vi "test_csm_helper2.vi"() -> ()   [LabVIEW 2020]
uses:
  <vilib>/Utility/traverseref.llb/TRef TravTarget.ctl
  <userlib>/_NEVSTOP/Communicable State Machine(CSM)/_Support/Priority Queue/Priority Queue.lvclass/Priority Queue.ctl
  Properties/Read VI Ref.vi
  <userlib>/_NEVSTOP/Communicable State Machine(CSM)/Utility/Build Error Cluster.vi
  <userlib>/_NEVSTOP/Communicable State Machine(CSM)/_Support/Process/CSMP-Sync Call.vi
  <userlib>/_NEVSTOP/Communicable State Machine(CSM)/Utility/uuid.vi
  <userlib>/_NEVSTOP/Communicable State Machine(CSM)/Utility/Trim Both Whitespace.vi
  <userlib>/_NEVSTOP/Communicable State Machine(CSM)/_Support/Process/CSMP-Async Call.vi
  <userlib>/_NEVSTOP/Communicable State Machine(CSM)/_Support/GlobalEvent/GEvt-Generate Status Log.vi
  <userlib>/_NEVSTOP/Communicable State Machine(CSM)/_Support/Process/CSMP-Broadcast.vi
  <userlib>/_NEVSTOP/Communicable State Machine(CSM)/_Support/GlobalEvent/GEvt-Generate Interrupt Log.vi
  <userlib>/_NEVSTOP/Communicable State Machine(CSM)/_Support/GlobalEvent/GEvt-Generate Register Log.vi
  <userlib>/_NEVSTOP/Communicable State Machine(CSM)/_Support/Process/CSMP-Register Status.vi
  <userlib>/_NEVSTOP/Communicable State Machine(CSM)/_Support/GlobalEvent/GEvt-Generate Unregister Log.vi
  <userlib>/_NEVSTOP/Communicable State Machine(CSM)/_Support/Process/CSMP-Unregister Status.vi
  <userlib>/_NEVSTOP/Communicable State Machine(CSM)/_Support/CSMQ/_CSMObj-Unlock.vi
  <userlib>/_NEVSTOP/Communicable State Machine(CSM)/_Support/Process/CSMP-PostPostMsg.vi
  <userlib>/_NEVSTOP/Communicable State Machine(CSM)/_Support/Process/CSMP-PostSendMsg.vi
  <userlib>/_NEVSTOP/Communicable State Machine(CSM)/_Support/CSMQ/_CSMObj-Lock State.vi
  <userlib>/_NEVSTOP/Communicable State Machine(CSM)/_Support/Common/Splite Reason String Part.vi
  <userlib>/_NEVSTOP/Communicable State Machine(CSM)/_Support/Common/Trim Single line Text.vi
  <userlib>/_NEVSTOP/Communicable State Machine(CSM)/_Support/CSMQ/_CSMOFGV Release.vi
  <userlib>/_NEVSTOP/Communicable State Machine(CSM)/_Support/Common/Remove Comments from Line.vi
  <userlib>/_NEVSTOP/Communicable State Machine(CSM)/_Support/Common/Splite Single-line Message.vi
  <userlib>/_NEVSTOP/Communicable State Machine(CSM)/_Support/Common/Parse Next Single-line State.vi
  <userlib>/_NEVSTOP/Communicable State Machine(CSM)/_Support/CSMQ/_CSMOFGV Dequeue.vi
  <userlib>/_NEVSTOP/Communicable State Machine(CSM)/_Support/CSMQ/_CSMObj-Log Error if in a Remote Session.vi
  <userlib>/_NEVSTOP/Communicable State Machine(CSM)/_Support/GlobalEvent/GEvt-Generate State Change Log.vi
  <userlib>/_NEVSTOP/Communicable State Machine(CSM)/_Support/GlobalEvent/GEvt-Generate Remaining States Log.vi
  <userlib>/_NEVSTOP/Communicable State Machine(CSM)/_Support/GlobalEvent/GEvt-Generate Module Destroyed Log.vi
  <userlib>/_NEVSTOP/Communicable State Machine(CSM)/_Support/GlobalEvent/GEvt-Generate Complete Log.vi
  <userlib>/_NEVSTOP/Communicable State Machine(CSM)/_Support/GlobalEvent/GEvt-Generate Module Created Log.vi
  <userlib>/_NEVSTOP/Communicable State Machine(CSM)/AdvanceAPI/CSM - Revert Arguments-Safe String.vi
  <userlib>/_NEVSTOP/Communicable State Machine(CSM)/AdvanceAPI/CSM - Make String Arguments Safe.vi
  <userlib>/_NEVSTOP/Communicable State Machine(CSM)/_Support/CSMQ/_CSMObj-Message Check.vi
  <userlib>/_NEVSTOP/Communicable State Machine(CSM)/_Support/CSMQ/_CSMObj-Enqueue Cross-Module Message.vi
  <userlib>/_NEVSTOP/Communicable State Machine(CSM)/_Support/CSMQ/_CSMOFGV Get.vi
  <userlib>/_NEVSTOP/Communicable State Machine(CSM)/_Support/FGV-BroadcastRegistry/Cache-Broadcast Registry Search Result.vi
  <userlib>/_NEVSTOP/Communicable State Machine(CSM)/AdvanceAPI/CSM - Register Status Change.vi
  <userlib>/_NEVSTOP/Communicable State Machine(CSM)/AdvanceAPI/CSM - Unregister Status Change.vi
  <userlib>/_NEVSTOP/Communicable State Machine(CSM)/_Support/Common/Hex Str to U8 Data.vi
  <userlib>/_NEVSTOP/Communicable State Machine(CSM)/_Support/Common/Concatenate State with Arguments.vi
  <userlib>/_NEVSTOP/Communicable State Machine(CSM)/_Support/Common/U8 Data to Hex Str.vi
  <userlib>/_NEVSTOP/Communicable State Machine(CSM)/_Support/Priority Queue/Dequeue Element.vi
  <userlib>/_NEVSTOP/Communicable State Machine(CSM)/AdvanceAPI/CSM - Keywords.vi
  <userlib>/_NEVSTOP/Communicable State Machine(CSM)/_Support/Priority Queue/Enqueue Element.vi
  <userlib>/_NEVSTOP/Communicable State Machine(CSM)/_Support/GlobalEvent/FGV-GlobalEventRef.vi
  <userlib>/_NEVSTOP/Communicable State Machine(CSM)/_Support/CSMQ/_CSMOFGV Obtain.vi
  <userlib>/_NEVSTOP/Communicable State Machine(CSM)/_Support/CSMQ/_CSMOFGV.vi
  <userlib>/_NEVSTOP/Communicable State Machine(CSM)/_Support/GlobalEvent/FGV-StatusChangeEventRef.vi
  <userlib>/_NEVSTOP/Communicable State Machine(CSM)/_Support/FGV-BroadcastRegistry/global-CSMQ FGV Change Flag.vi
  <userlib>/_NEVSTOP/Communicable State Machine(CSM)/_Support/FGV-BroadcastRegistry/global-Broadcast Cache Change Flag.vi
  <userlib>/_NEVSTOP/Communicable State Machine(CSM)/_Support/BroadcastRegistry/HelperVI/Broadcast Item Key.vi
  <userlib>/_NEVSTOP/Communicable State Machine(CSM)/_Support/FGV-BroadcastRegistry/FGV-BroadcastRegistry.vi
  <userlib>/_NEVSTOP/Communicable State Machine(CSM)/_Support/Message/Parse Register Message.vi
  <userlib>/_NEVSTOP/Communicable State Machine(CSM)/_Support/Message/Parse Unregister Message.vi
  API/Create From VI Reference.vi
  API/Destroy.vi
  <userlib>/_NEVSTOP/Communicable State Machine(CSM)/Communicable State Machine.lvlib
  CSM-Helper.lvclass
  <vilib>/Utility/traverseref.llb/VI Scripting - Traverse.lvlib
  34952832-c283-4153-b183-f70f505a0969.vi
panel:
  out "Array":path[](array[path])
  out "State History":string
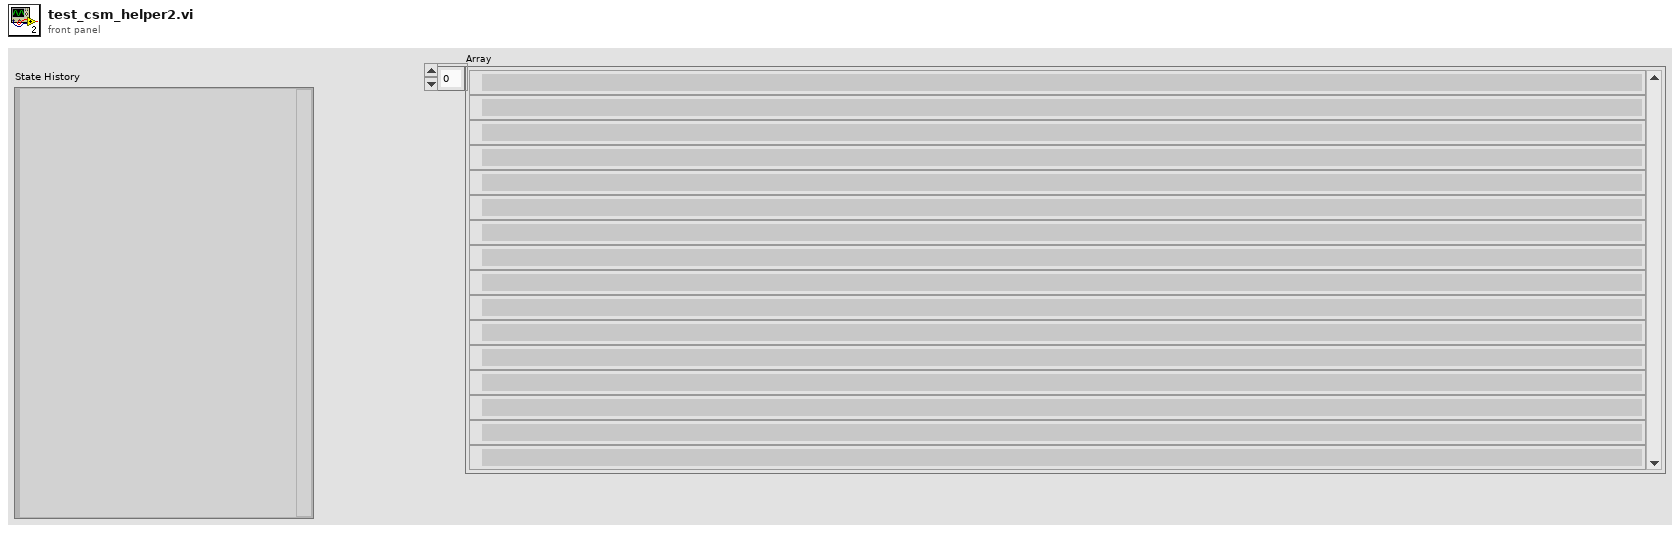
[diagram p1: front panel]
types:
  T1 = typedef "TRef TravTarget.ctl" = enum16{"FP", "BD", "Other"}
  T2 = enum32{"Invalid", "Standard", "Closed", "Hidden", "Minimized", "Maximized"}
  T3 = enum32{"invalid app kind", "Development System", "Run Time System", "Student Edition", "Embedded LabVIEW", "Evaluation", "Custom"}
  T4 = typedef "Communicable State Machine.lvlib/_CSM_Response Source Message.ctl" = cluster{"‘State":string, "’Arguments":string, "’Error":errorcluster}
  T5 = cluster{"Core":cluster{"Current VI Reference":refnum<vi>, "Close Panel on Exit?":bool}, "Your Boolean data":bool, "Your string data":string}
  T6 = cluster{"Current VI Reference":refnum<vi>, "Close Panel on Exit?":bool}
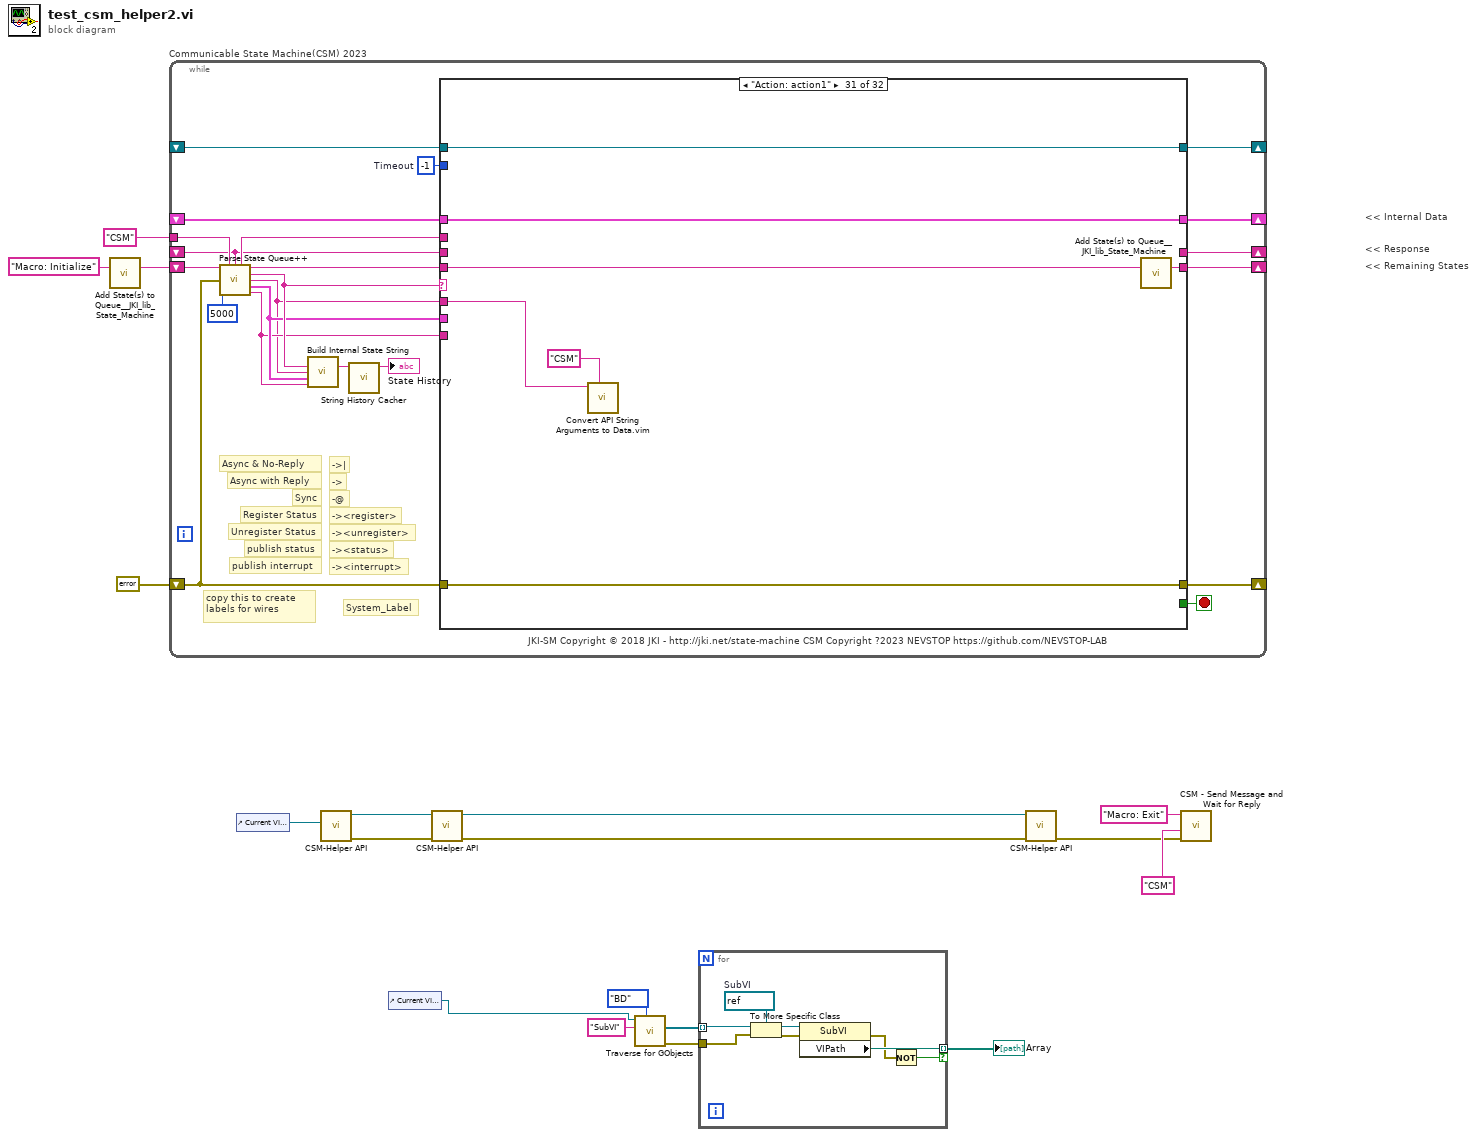
[diagram p0: block diagram]
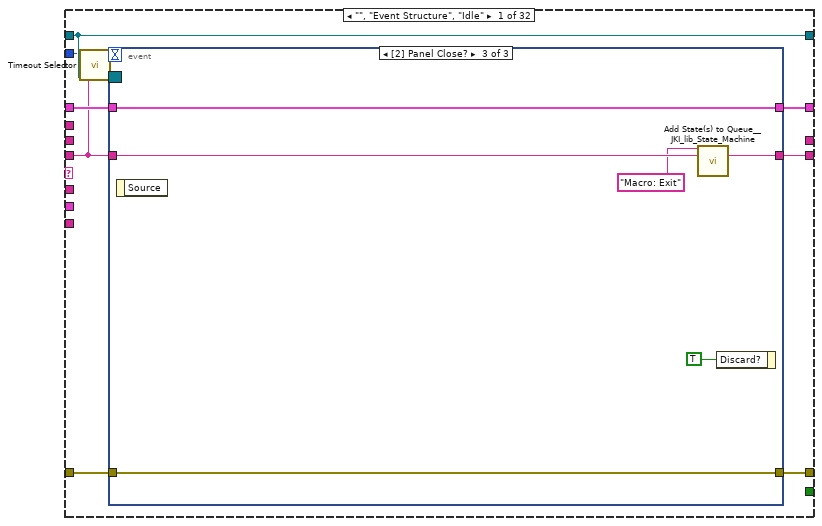
[diagram p2: hidden frame]
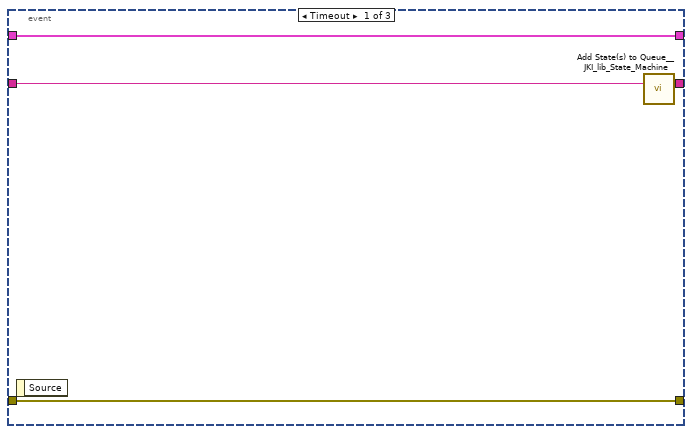
[diagram p3: hidden frame]
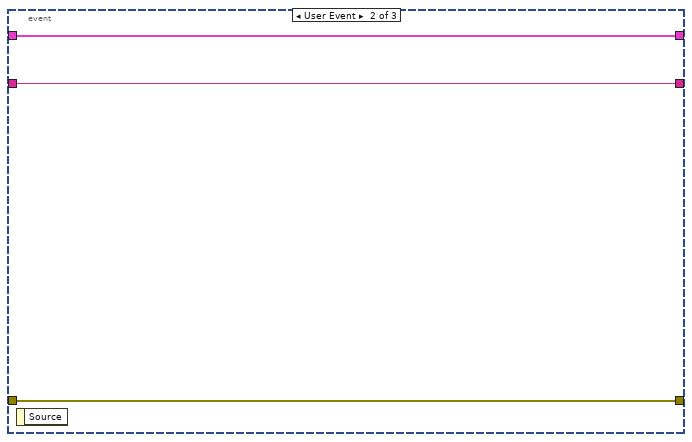
[diagram p4: hidden frame]
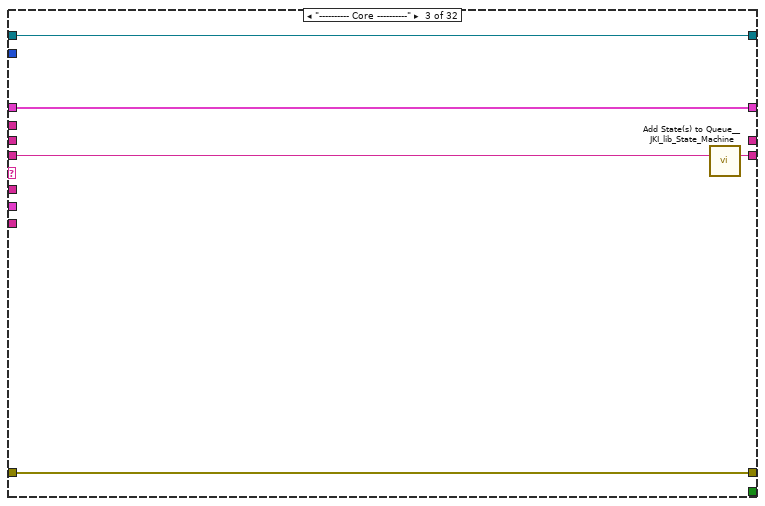
[diagram p6: hidden frame]
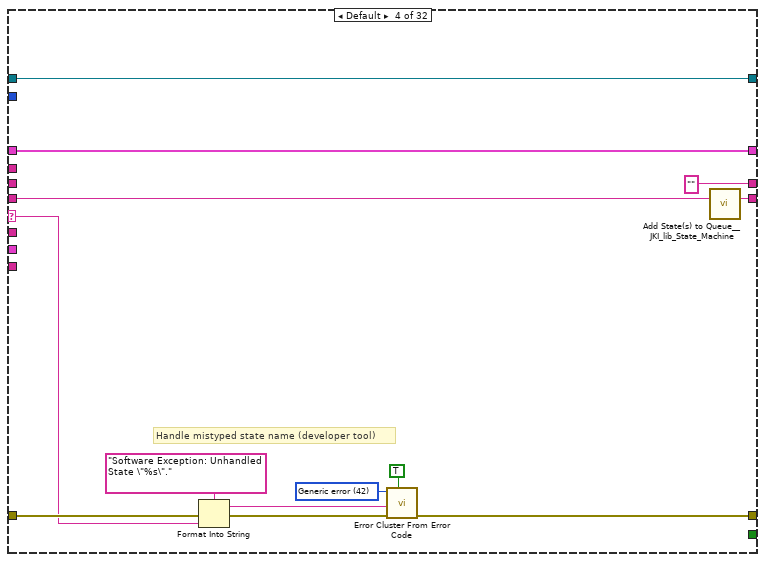
[diagram p7: hidden frame]
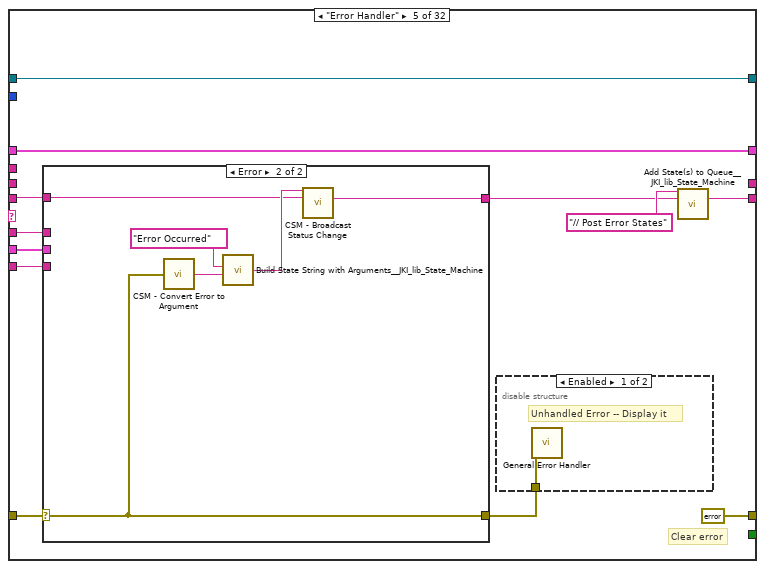
[diagram p8: hidden frame]
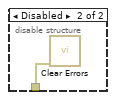
[diagram p9: hidden frame]
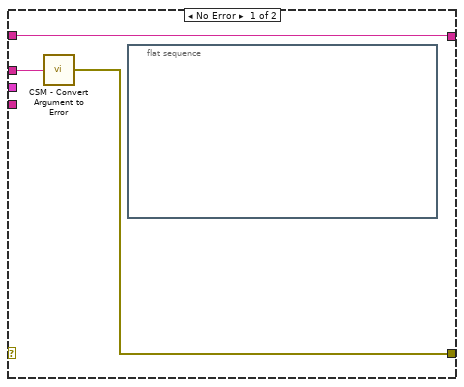
[diagram p10: hidden frame]
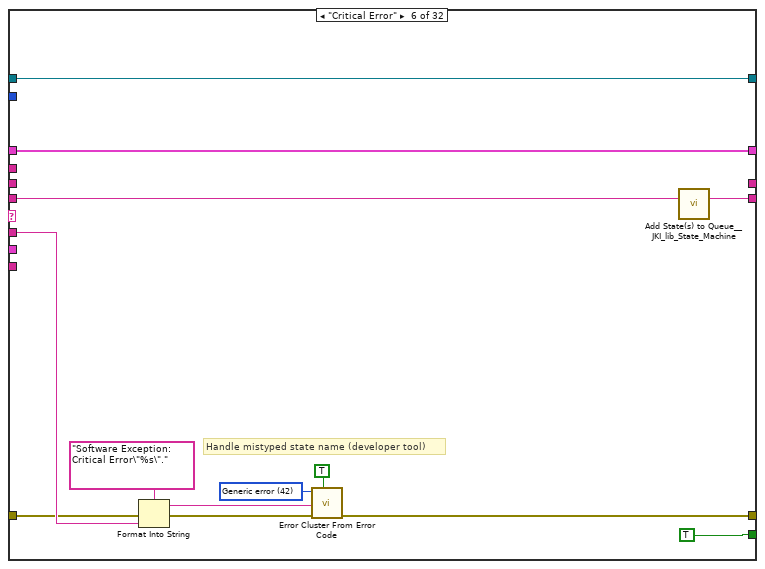
[diagram p11: hidden frame]
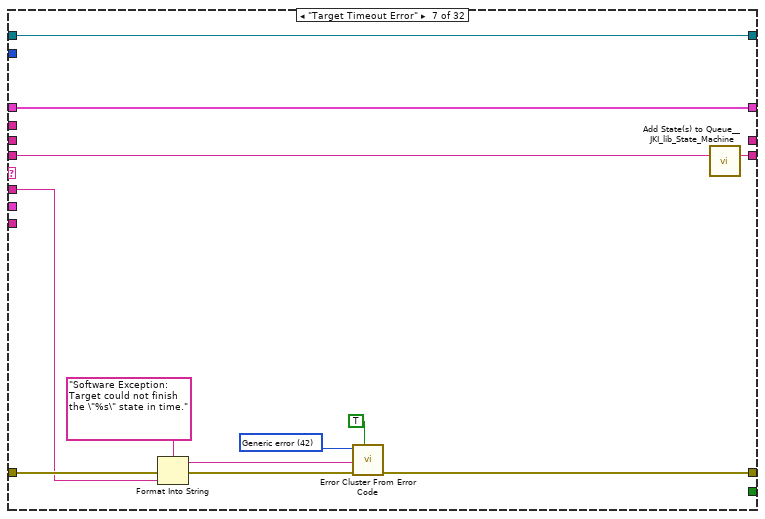
[diagram p12: hidden frame]
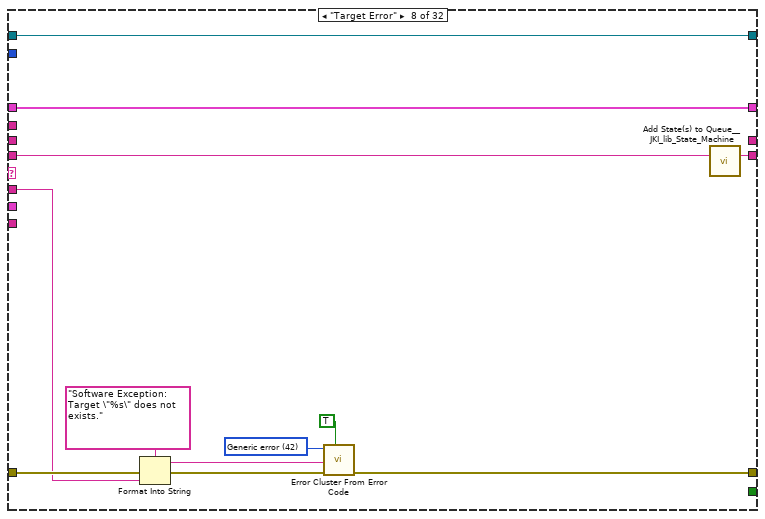
[diagram p13: hidden frame]
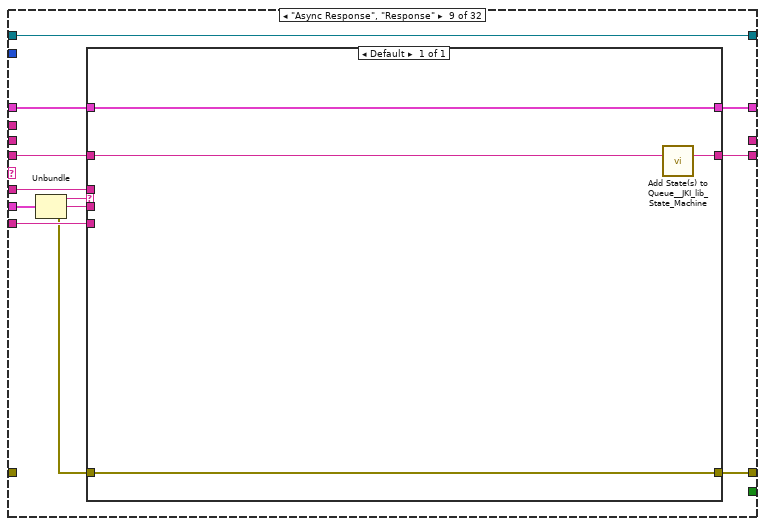
[diagram p14: hidden frame]
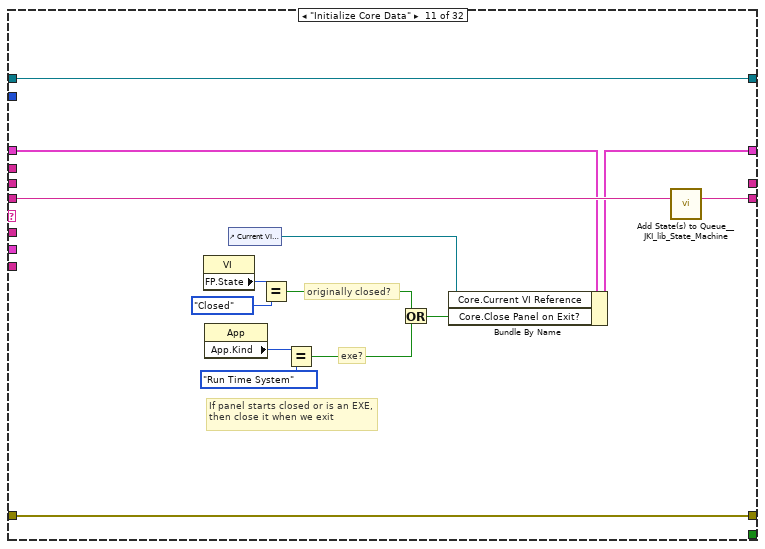
[diagram p16: hidden frame]
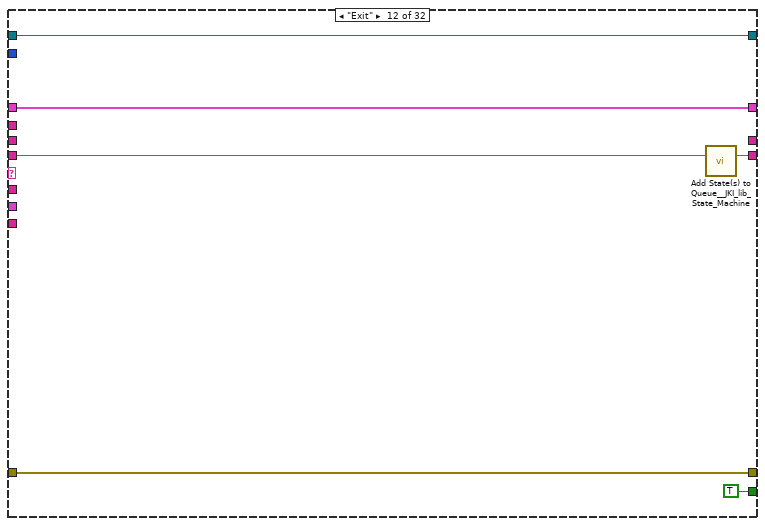
[diagram p17: hidden frame]
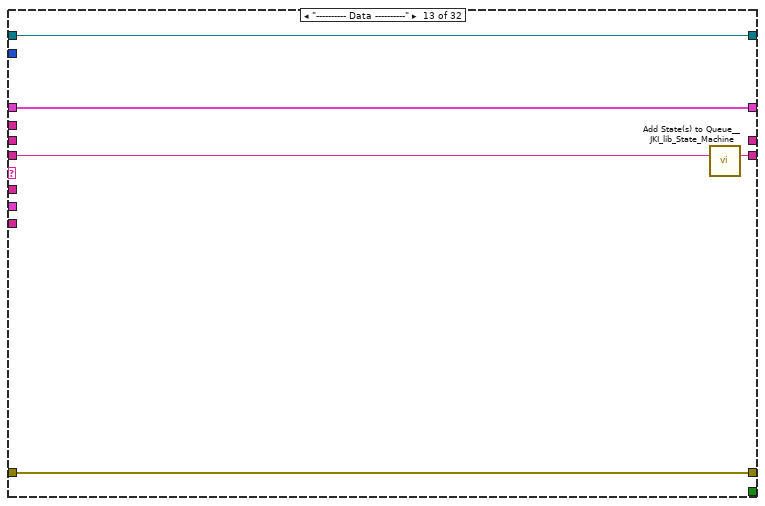
[diagram p18: hidden frame]
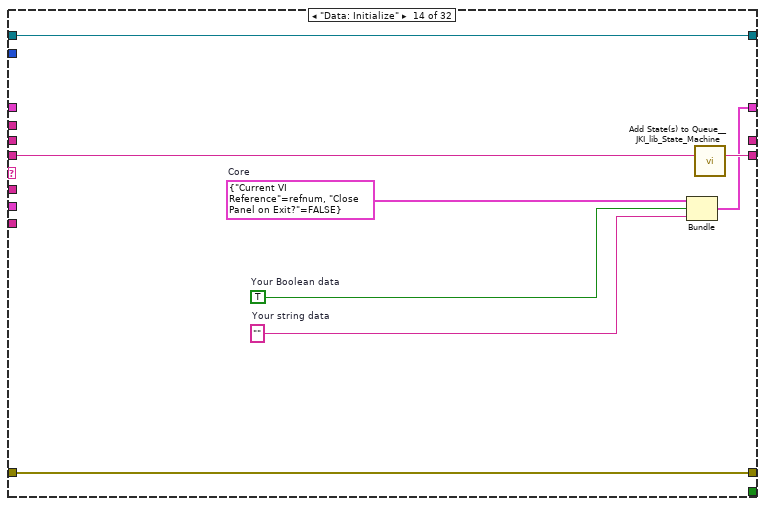
[diagram p19: hidden frame]
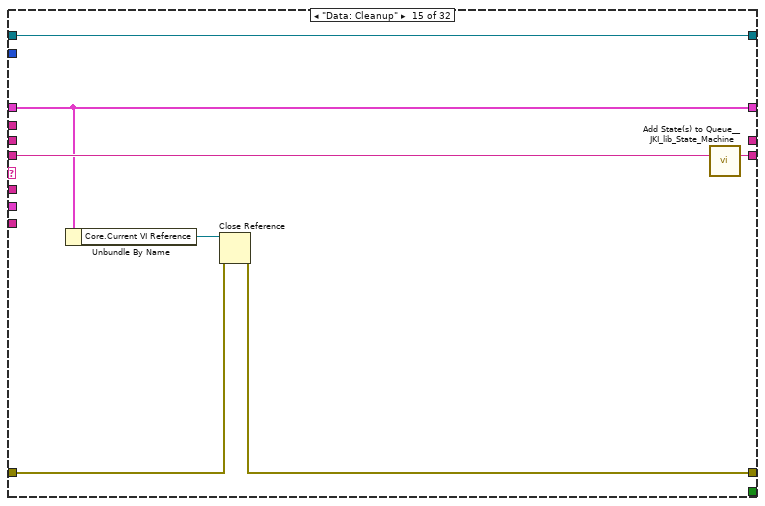
[diagram p20: hidden frame]
diagram:
  # "<< Internal Data"
  # "<< Response"
  # "<< Remaining States"
  n1 = call <vilib>:"Add State(s) to Queue__JKI_lib_State_Machine.vi"("State(s) in (\"\")"="Macro: Initialize" ("Init State(\"Macro: Initialize\")")) -> ("States Out"=w15:string)  [unwired: 14 in]
  n2 = while "Communicable State Machine(CSM) 2023" {
    shift-right: [w35] -> _
    shift-left: _ -> [w34]
    shift-right: [w38] -> _
    shift-left: errorcluster {"status"=FALSE, "code"=0, "source"=""} ("error out") -> [w32]
    shift-right: [w37] -> _
    shift-left: w15 -> [w39]
    tunnel: "CSM" ("Name(\"\" to use uuid)") -> [w27]
    shift-right: [w30] -> _
    shift-left: _ -> [w20]
    shift-right: [w29] -> _
    shift-left: _ -> [w28]
    stop <- w36 stop-if-true
    w33 = -1  # Timeout
    # "-><interrupt>"
    # "-><status>"
    # "-><unregister>"
    # "-><register>"
    # "-@"
    # "->"
    # "->|"
    # "publish interrupt"
    # "publish status"
    # "Unregister Status"
    # "Register Status"
    # "Sync"
    # "Async with Reply"
    # "Async & No-Reply"
    # "copy this to create labels for wires"
    # "System_Label"
    # "JKI-SM Copyright © 2018 JKI - http://jki.net/state-machine CSM Copyright ?2023 NEVSTOP https://github.com/NEVSTOP-LAB"
    n3 = call <userlib>:"Parse State Queue++.vi"("State Queue"=w39, "Name(\"\" to use uuid)"=w27, "Response Arguments"=w20, "Error In (no error)"=w32, "Response Timeout(5000ms)"=5000 ("Response Timeout(1000ms)")) -> ("Name Used"=w21:string, "Remaining States"=w40:string, "Current State"=w24:string, "Arguments"=w19:string, ">> Response Source Message >>"=w23:T4, ">> Source CSM >>"=w22:string)  [unwired: 5 in]
    n4 = call <userlib>:"Build Internal State String.vi"("State"=w24, "Arguments (\"\")"=w19, ">> Response Source Message >>"=w23, "Source (\"\")"=w22) -> ("State with Arguments"=w25:string)  [unwired: 11 in]
    n5 = call <userlib>:"String History Cacher.vi"("String"=w25) -> ("String Cache"=→"State History":string)  [unwired: 10 in]
    n6 = case shown="\"Action: action1\"" w24 {
      selector: w24 -> [_ _ _ w74 _ _ _ _ _ _ _ _ _ _ _ _ _ _ _ _ _ _ _ _ _ _ _ _ _ _ _ _]
      tunnel: w40 -> [w41 w66 w71 w78 w89 w119 w127 w139 w154 w163 w178 w184 w189 w197 w204 w209 w216 w220 w226 w231 w238 w254 w324 w330 w342 w345 w351 w355 w359 w366 w373 w378]
      tunnel: w19 -> [_ _ _ _ w87 w112 w123 w135 w148 _ _ _ _ _ _ _ _ _ _ _ w233 w248 _ _ _ _ w347 _ _ _ w368 _]
      tunnel: w34 -> [w48 w65 w68 w76 w95 w120 w125 w137 w152 w162 w171 w182 w186 _ w199 w206 w215 w219 w223 w229 w236 w250 w321 w327 w339 w344 w350 w354 w358 w363 w370 w375]
      tunnel: [w47 w64 w69 w80 errorcluster {"status"=FALSE, "code"=0, "source"=""} ("error out") w108 w121 w133 w151 w164 w175 w181 w187 w194 w200 w207 w210 w218 w224 w228 w234 w251 w322 w328 w340 w346 w352 w356 w360 w364 w371 w376] -> w38
      tunnel: w32 -> [w46 w64 w69 w79 w93 w109 w128 w140 _ w164 w175 w181 w187 w194 w201 w207 _ w221 w224 w228 w235 w252 w322 w328 w340 w346 w352 w356 w360 w364 w371 w376]
      tunnel: [w49 w66 w70 w77 w91 w118 w126 w138 w155 w163 w177 w183 w188 w196 w203 w208 w216 w220 w225 w230 w237 w253 w323 w329 w341 w345 w351 w355 w359 w365 w372 w377] -> w37
      tunnel: [_ _ _ _ _ TRUE _ _ _ _ _ TRUE _ _ _ _ _ _ _ _ _ _ _ _ _ _ _ _ _ _ _ _] -> w36
      tunnel: [w45 w65 w68 w76 w95 w120 w125 w137 w153 w162 w176 w182 w186 w195 w199 w206 w215 w219 w223 w229 w236 w250 w321 w327 w339 w344 w350 w354 w358 w363 w370 w375] -> w35
      tunnel: w33 -> [w43 _ _ _ _ _ _ _ _ _ _ _ _ _ _ _ _ _ _ _ _ _ _ _ _ _ _ _ _ _ _ _]
      tunnel: w22 -> [_ _ _ _ w86 _ _ _ w149 _ _ _ _ _ _ _ _ _ _ _ _ _ _ _ _ _ _ _ _ _ _ _]
      tunnel: w23 -> [_ _ _ _ w85 _ _ _ w150 _ _ _ _ _ _ _ _ _ _ _ _ _ _ _ _ _ _ _ _ _ _ _]
      tunnel: [_ _ _ "" _ _ _ _ _ _ _ _ _ _ _ _ _ _ _ _ _ _ _ _ _ _ "API1 Response" _ _ _ _ _] -> w30
      tunnel: [w44 w63 w67 w72 w94 w110 w122 w134 w156 w161 w165 w179 w185 w190 w198 w205 w214 w217 w222 w227 w232 w247 w320 w325 w332 w343 w349 w353 w357 w362 w369 w374] -> w29
      tunnel: w28 -> [w44 w63 w67 w72 w94 w110 w122 w134 w156 w161 w165 w179 w185 w190 w198 w205 _ w217 w222 w227 w232 w247 w320 w325 w332 w343 w349 w353 w357 w362 w369 w374]
      tunnel: w21 -> [_ _ _ _ _ _ _ _ _ _ _ _ _ _ _ _ w213 _ _ _ _ _ _ _ _ _ _ _ _ _ _ _]
      tunnel: w20 -> [_ _ _ _ _ _ _ _ _ _ _ _ _ _ _ _ _ _ _ _ _ _ _ _ _ _ _ _ _ _ _ _]
      frame "", "Event Structure", "Idle" {
        n7 = call <userlib>:"Timeout Selector.vi"("Remaining States"=w41, "Timeout Expected"=w43) -> ("Timeout"=w42:i32)  [unwired: 5 in]
        n8 = event shown="[2] Panel Close?" {
          selector: w44 -> [_ _ _]
          dyn-events: _ -> [_ _ _]
          timeout: w42 -> [_ _ _]
          tunnel: w41 -> [w53 w55 w62]
          tunnel: [w52 w55 w61] -> w49
          tunnel: w48 -> [w50 w56 w59]
          tunnel: [w51 w54 w60] -> w47
          tunnel: w46 -> [w51 w54 w60]
          tunnel: [w50 w56 w59] -> w45
          event Timeout {
            n9 = event-data() -> ()  [unwired: 1 in, 1 out]
            n10 = call <vilib>:"Add State(s) to Queue__JKI_lib_State_Machine.vi"("State(s) in (\"\")"=w53) -> ("States Out"=w52:string)  [unwired: 14 in]
          }
          event User Event {
            n11 = event-data() -> ()  [unwired: 1 in, 1 out]
          }
          event Panel Close? {
            n12 = event-data() -> ()  [unwired: 1 in, 1 out]
            n13 = call <vilib>:"Add State(s) to Queue__JKI_lib_State_Machine.vi"("State(s) in Front (\"\")"="Macro: Exit", "State(s) in (\"\")"=w62) -> ("States Out"=w61:string)  [unwired: 13 in]
            n14 = event-data("Discard?"=TRUE) -> ()  [unwired: 1 in, 1 out]
          }
        }
      }
      frame "CSM Documentation" {
      }
      frame "---------- Core ----------" {
        n15 = call <vilib>:"Add State(s) to Queue__JKI_lib_State_Machine.vi"("State(s) in (\"\")"=w71) -> ("States Out"=w70:string)  [unwired: 14 in]
      }
      frame Default {
        w83 = 42 items=["No error", "Argument error", "Memory is full", "Out of zone", "End of file", "File already open", "Generic file I/O error", "File not found", "File permission error", "Disk is full", "Duplicate path", "Too many files open", "System feature not enabled", "Resource file not found", "Cannot add resource", "Resource not found", "Image not found", "Image memory error", "Pen does not exist", "Config type invalid", "Config token not found", "Config parse error", "Config memory error", "Bad external code format", "Bad external code offset", "External code not present", "Null window", "Destroy window error", "Null menu", "Print aborted", "Bad print record", "Print driver error", "Windows error during printing", "Memory error during printing", "Print dialog error", "Generic print error", "Invalid device refnum", "Device not found", "Device parameter error", "Device unit error", "Cannot open device", "Device call aborted", "Generic error", "Cancelled by user", "Object ID too low", "Object ID too high", "Object not in heap", "Unknown heap", "Unknown object (invalid DefProc)", "Unknown object (DefProc not in table)", "Message out of range", "Invalid (null) method", "Unknown message", "Manager call not supported", "Bad address", "Network operation in progress", "Network operation timed out", "Connection is busy", "Network attribute not supported", "Network error", "Address in use", "System out of memory", "Connection aborted", "Connection refused", "Not connected", "Already connected", "Connection closed", "Initialization error (interapplication manager)", "Bad occurrence", "Wait on unbound occurrence handler", "Occurrence queue overflow", "Datalog type conflict", "Unused", "Unrecognized type (interapplication manager)", "Memory corrupt", "Failed to make temporary DLL", "Old CIN version", "Drag socket not found", "Failed to load drop-object", "Failed to register OLE object", "Failed to release OLE object", "Format specifier type mismatch", "Unknown format specifier", "Too few format specifiers", "Too many format specifiers", "Scan failed", "Newer CIN version", "Error converting to variant", "Runtime menu error", "Password tampered", "Variant attribute not found", "Incompatible variant data type", "Event data is not available", "Event Store is not present", "Occurrence is not found", "Event Queue is not created", "Event info is not available", "Refnum passed is NULL", "Error retrieving Class GUID", "Error retrieving CoClass GUID", "Error retrieving TypeLib GUID.", "Bad built application magic bytes.", "Specific driver is different from the specific driver associated with the Logical Name.", "There is no session opened to the class driver.", "Max Error", "MAX - Error with config objects", "MAX - Error loading configuration", "MAX - Group not supported"]
        # "Handle mistyped state name (developer tool)"
        n16 = Format Into String(format string="Software Exception: Unhandled State \"%s\"." ("message"), error in=w79, w74) -> (resulting string=w82:string, error out=w81:errorcluster)  [unwired: 1 in]
        n17 = call <vilib>:"Error Cluster From Error Code.vi"("show call chain? (False)"=TRUE, "error in (no error)"=w81, "error message (\"\")"=w82, "error code (0)"=w83) -> ("error out"=w80:errorcluster)  [unwired: 5 in]
        n18 = call <vilib>:"Add State(s) to Queue__JKI_lib_State_Machine.vi"("State(s) in (\"\")"=w78) -> ("States Out"=w77:string)  [unwired: 14 in]
      }
      frame "Error Handler" {
        # "Clear error"
        n19 = case shown="Error" w93 {
          selector: w93 -> [_ w102]
          tunnel: [w100 w104] -> w90
          tunnel: w89 -> [w100 w103]
          tunnel: [w99 w102] -> w88
          tunnel: w87 -> [w101 _]
          tunnel: w86 -> [_ _]
          tunnel: w85 -> [_ _]
          frame No Error {
            n20 = call <userlib>:"CSM - Convert Argument to Error.vi"("Argument"=w101) -> ("error"=w99:errorcluster)  [unwired: 4 in]
            n21 = flat-sequence {
              frame #0 {
              }
            }
          }
          frame Error {
            n22 = call <userlib>:"CSM - Convert Error to Argument.vi"("error in (no error)"=w102) -> ("Arguments"=w106:string)  [unwired: 4 in]
            n23 = call <vilib>:"Build State String with Arguments__JKI_lib_State_Machine.vi"("Arguments (\"\")"=w106, "State"="Error Occurred" ("Status with Arguments")) -> ("State with Arguments"=w105:string)  [unwired: 4 in]
            n24 = call <userlib>:"CSM - Broadcast Status Change.vi"("Status with Arguments"=w105, "State Queue"=w103) -> ("Remaining States"=w104:string)  [unwired: 13 in]
          }
        }
        n25 = disable-structure shown="Enabled" {
          disable-tunnel: w88 -> [w97 w98]
          frame Enabled {
            # "Unhandled Error -- Display it"
            n26 = call <vilib>:"General Error Handler.vi"("error in (no error)"=w97) -> ()  [unwired: 10 in, 5 out]
          }
          frame Disabled {
            n27 = call <vilib>:"Clear Errors.vi"("error in (no error)"=w98) -> ()  [unwired: 5 in, 2 out]
          }
        }
        n28 = call <vilib>:"Add State(s) to Queue__JKI_lib_State_Machine.vi"("State(s) in Front (\"\")"="// Post Error States", "State(s) in (\"\")"=w90) -> ("States Out"=w91:string)  [unwired: 13 in]
      }
      frame "Critical Error" {
        w116 = 42 items=["No error", "Argument error", "Memory is full", "Out of zone", "End of file", "File already open", "Generic file I/O error", "File not found", "File permission error", "Disk is full", "Duplicate path", "Too many files open", "System feature not enabled", "Resource file not found", "Cannot add resource", "Resource not found", "Image not found", "Image memory error", "Pen does not exist", "Config type invalid", "Config token not found", "Config parse error", "Config memory error", "Bad external code format", "Bad external code offset", "External code not present", "Null window", "Destroy window error", "Null menu", "Print aborted", "Bad print record", "Print driver error", "Windows error during printing", "Memory error during printing", "Print dialog error", "Generic print error", "Invalid device refnum", "Device not found", "Device parameter error", "Device unit error", "Cannot open device", "Device call aborted", "Generic error", "Cancelled by user", "Object ID too low", "Object ID too high", "Object not in heap", "Unknown heap", "Unknown object (invalid DefProc)", "Unknown object (DefProc not in table)", "Message out of range", "Invalid (null) method", "Unknown message", "Manager call not supported", "Bad address", "Network operation in progress", "Network operation timed out", "Connection is busy", "Network attribute not supported", "Network error", "Address in use", "System out of memory", "Connection aborted", "Connection refused", "Not connected", "Already connected", "Connection closed", "Initialization error (interapplication manager)", "Bad occurrence", "Wait on unbound occurrence handler", "Occurrence queue overflow", "Datalog type conflict", "Unused", "Unrecognized type (interapplication manager)", "Memory corrupt", "Failed to make temporary DLL", "Old CIN version", "Drag socket not found", "Failed to load drop-object", "Failed to register OLE object", "Failed to release OLE object", "Format specifier type mismatch", "Unknown format specifier", "Too few format specifiers", "Too many format specifiers", "Scan failed", "Newer CIN version", "Error converting to variant", "Runtime menu error", "Password tampered", "Variant attribute not found", "Incompatible variant data type", "Event data is not available", "Event Store is not present", "Occurrence is not found", "Event Queue is not created", "Event info is not available", "Refnum passed is NULL", "Error retrieving Class GUID", "Error retrieving CoClass GUID", "Error retrieving TypeLib GUID.", "Bad built application magic bytes.", "Specific driver is different from the specific driver associated with the Logical Name.", "There is no session opened to the class driver.", "Max Error", "MAX - Error with config objects", "MAX - Error loading configuration", "MAX - Group not supported"]
        # "Handle mistyped state name (developer tool)"
        n29 = Format Into String(format string="Software Exception: Critical Error\"%s\"." ("message"), error in=w109, w112) -> (resulting string=w115:string, error out=w114:errorcluster)  [unwired: 1 in]
        n30 = call <vilib>:"Error Cluster From Error Code.vi"("show call chain? (False)"=TRUE, "error in (no error)"=w114, "error message (\"\")"=w115, "error code (0)"=w116) -> ("error out"=w108:errorcluster)  [unwired: 5 in]
        n31 = call <vilib>:"Add State(s) to Queue__JKI_lib_State_Machine.vi"("State(s) in (\"\")"=w119) -> ("States Out"=w118:string)  [unwired: 14 in]
      }
      frame "Target Timeout Error" {
        w131 = 42 items=["No error", "Argument error", "Memory is full", "Out of zone", "End of file", "File already open", "Generic file I/O error", "File not found", "File permission error", "Disk is full", "Duplicate path", "Too many files open", "System feature not enabled", "Resource file not found", "Cannot add resource", "Resource not found", "Image not found", "Image memory error", "Pen does not exist", "Config type invalid", "Config token not found", "Config parse error", "Config memory error", "Bad external code format", "Bad external code offset", "External code not present", "Null window", "Destroy window error", "Null menu", "Print aborted", "Bad print record", "Print driver error", "Windows error during printing", "Memory error during printing", "Print dialog error", "Generic print error", "Invalid device refnum", "Device not found", "Device parameter error", "Device unit error", "Cannot open device", "Device call aborted", "Generic error", "Cancelled by user", "Object ID too low", "Object ID too high", "Object not in heap", "Unknown heap", "Unknown object (invalid DefProc)", "Unknown object (DefProc not in table)", "Message out of range", "Invalid (null) method", "Unknown message", "Manager call not supported", "Bad address", "Network operation in progress", "Network operation timed out", "Connection is busy", "Network attribute not supported", "Network error", "Address in use", "System out of memory", "Connection aborted", "Connection refused", "Not connected", "Already connected", "Connection closed", "Initialization error (interapplication manager)", "Bad occurrence", "Wait on unbound occurrence handler", "Occurrence queue overflow", "Datalog type conflict", "Unused", "Unrecognized type (interapplication manager)", "Memory corrupt", "Failed to make temporary DLL", "Old CIN version", "Drag socket not found", "Failed to load drop-object", "Failed to register OLE object", "Failed to release OLE object", "Format specifier type mismatch", "Unknown format specifier", "Too few format specifiers", "Too many format specifiers", "Scan failed", "Newer CIN version", "Error converting to variant", "Runtime menu error", "Password tampered", "Variant attribute not found", "Incompatible variant data type", "Event data is not available", "Event Store is not present", "Occurrence is not found", "Event Queue is not created", "Event info is not available", "Refnum passed is NULL", "Error retrieving Class GUID", "Error retrieving CoClass GUID", "Error retrieving TypeLib GUID.", "Bad built application magic bytes.", "Specific driver is different from the specific driver associated with the Logical Name.", "There is no session opened to the class driver.", "Max Error", "MAX - Error with config objects", "MAX - Error loading configuration", "MAX - Group not supported"]
        n32 = Format Into String(format string="Software Exception: Target could not finish the \"%s\" state in time." ("message"), error in=w128, w123) -> (resulting string=w130:string, error out=w129:errorcluster)  [unwired: 1 in]
        n33 = call <vilib>:"Error Cluster From Error Code.vi"("show call chain? (False)"=TRUE, "error in (no error)"=w129, "error message (\"\")"=w130, "error code (0)"=w131) -> ("error out"=w121:errorcluster)  [unwired: 5 in]
        n34 = call <vilib>:"Add State(s) to Queue__JKI_lib_State_Machine.vi"("State(s) in (\"\")"=w127) -> ("States Out"=w126:string)  [unwired: 14 in]
      }
      frame "Target Error" {
        w143 = 42 items=["No error", "Argument error", "Memory is full", "Out of zone", "End of file", "File already open", "Generic file I/O error", "File not found", "File permission error", "Disk is full", "Duplicate path", "Too many files open", "System feature not enabled", "Resource file not found", "Cannot add resource", "Resource not found", "Image not found", "Image memory error", "Pen does not exist", "Config type invalid", "Config token not found", "Config parse error", "Config memory error", "Bad external code format", "Bad external code offset", "External code not present", "Null window", "Destroy window error", "Null menu", "Print aborted", "Bad print record", "Print driver error", "Windows error during printing", "Memory error during printing", "Print dialog error", "Generic print error", "Invalid device refnum", "Device not found", "Device parameter error", "Device unit error", "Cannot open device", "Device call aborted", "Generic error", "Cancelled by user", "Object ID too low", "Object ID too high", "Object not in heap", "Unknown heap", "Unknown object (invalid DefProc)", "Unknown object (DefProc not in table)", "Message out of range", "Invalid (null) method", "Unknown message", "Manager call not supported", "Bad address", "Network operation in progress", "Network operation timed out", "Connection is busy", "Network attribute not supported", "Network error", "Address in use", "System out of memory", "Connection aborted", "Connection refused", "Not connected", "Already connected", "Connection closed", "Initialization error (interapplication manager)", "Bad occurrence", "Wait on unbound occurrence handler", "Occurrence queue overflow", "Datalog type conflict", "Unused", "Unrecognized type (interapplication manager)", "Memory corrupt", "Failed to make temporary DLL", "Old CIN version", "Drag socket not found", "Failed to load drop-object", "Failed to register OLE object", "Failed to release OLE object", "Format specifier type mismatch", "Unknown format specifier", "Too few format specifiers", "Too many format specifiers", "Scan failed", "Newer CIN version", "Error converting to variant", "Runtime menu error", "Password tampered", "Variant attribute not found", "Incompatible variant data type", "Event data is not available", "Event Store is not present", "Occurrence is not found", "Event Queue is not created", "Event info is not available", "Refnum passed is NULL", "Error retrieving Class GUID", "Error retrieving CoClass GUID", "Error retrieving TypeLib GUID.", "Bad built application magic bytes.", "Specific driver is different from the specific driver associated with the Logical Name.", "There is no session opened to the class driver.", "Max Error", "MAX - Error with config objects", "MAX - Error loading configuration", "MAX - Group not supported"]
        n35 = Format Into String(format string="Software Exception: Target \"%s\" does not exists." ("message"), error in=w140, w135) -> (resulting string=w142:string, error out=w141:errorcluster)  [unwired: 1 in]
        n36 = call <vilib>:"Error Cluster From Error Code.vi"("show call chain? (False)"=TRUE, "error in (no error)"=w141, "error message (\"\")"=w142, "error code (0)"=w143) -> ("error out"=w133:errorcluster)  [unwired: 5 in]
        n37 = call <vilib>:"Add State(s) to Queue__JKI_lib_State_Machine.vi"("State(s) in (\"\")"=w139) -> ("States Out"=w138:string)  [unwired: 14 in]
      }
      frame "Async Response", "Response" {
        n38 = Unbundle(w150) -> ("‘State"=w147:string, "’Arguments"=w146:string, "’Error"=w145:errorcluster)
        n39 = case shown="Default" w147 {
          tunnel: [w157] -> w155
          tunnel: w154 -> [w158]
          tunnel: [w160] -> w153
          tunnel: w152 -> [w160]
          tunnel: [w159] -> w151
          tunnel: w145 -> [w159]
          tunnel: w149 -> [_]
          tunnel: w148 -> [_]
          tunnel: w146 -> [_]
          frame Default {
            n40 = call <vilib>:"Add State(s) to Queue__JKI_lib_State_Machine.vi"("State(s) in (\"\")"=w158) -> ("States Out"=w157:string)  [unwired: 14 in]
          }
        }
      }
      frame "Async Message Posted" {
      }
      frame "Initialize Core Data" {
        # "originally closed?"
        # "exe?"
        # "If panel starts closed or is an EXE, then close it when we exit"
        n41 = property class="VI"() -> ("FP.State"=w168:T2)  [unwired: 2 in, 2 out]
        n42 = property class="App"() -> ("App.Kind"=w174:T3)  [unwired: 2 in, 2 out]
        n43 = control-ref of="Current VI Reference"() -> (w169:refnum<vi>)
        n44 = Equal?(x=w168, y=T2."Closed" ("Front Panel Window:State")) -> (x = y?=w166:bool)
        n45 = Equal?(x=w174, y=T3."Run Time System" ("Application:Kind")) -> (x = y?=w172:bool)
        n46 = Or(x=w166, y=w172) -> (x .or. y?=w170:bool)
        n47 = Bundle By Name(cluster=w171, "Core.Current VI Reference"=w169, "Core.Close Panel on Exit?"=w170) -> (w176:T5)
        n48 = call <vilib>:"Add State(s) to Queue__JKI_lib_State_Machine.vi"("State(s) in (\"\")"=w178) -> ("States Out"=w177:string)  [unwired: 14 in]
      }
      frame "Exit" {
        n49 = call <vilib>:"Add State(s) to Queue__JKI_lib_State_Machine.vi"("State(s) in (\"\")"=w184) -> ("States Out"=w183:string)  [unwired: 14 in]
      }
      frame "---------- Data ----------" {
        n50 = call <vilib>:"Add State(s) to Queue__JKI_lib_State_Machine.vi"("State(s) in (\"\")"=w189) -> ("States Out"=w188:string)  [unwired: 14 in]
      }
      frame "Data: Initialize" {
        w191 = T6 {"Current VI Reference"=refnum, "Close Panel on Exit?"=FALSE}  # Core
        w193 = TRUE  # Your Boolean data
        w192 = ""  # Your string data
        n51 = Bundle("Core"=w191, "Your Boolean data"=w193, "Your string data"=w192) -> (w195:T5)  [unwired: 1 in]
        n52 = call <vilib>:"Add State(s) to Queue__JKI_lib_State_Machine.vi"("State(s) in (\"\")"=w197) -> ("States Out"=w196:string)  [unwired: 14 in]
      }
      frame "Data: Cleanup" {
        n53 = Unbundle By Name(w199) -> ("Core.Current VI Reference"=w202:refnum<vi>)
        n54 = Close Reference(reference=w202, error in (no error)=w201) -> (error out=w200:errorcluster)
        n55 = call <vilib>:"Add State(s) to Queue__JKI_lib_State_Machine.vi"("State(s) in (\"\")"=w204) -> ("States Out"=w203:string)  [unwired: 14 in]
      }
      frame "---------- Events ----------" {
        n56 = call <vilib>:"Add State(s) to Queue__JKI_lib_State_Machine.vi"("State(s) in (\"\")"=w209) -> ("States Out"=w208:string)  [unwired: 14 in]
      }
      frame "Events: Register" {
        n57 = call <userlib>:"CSM - Get New State Notifier Event.vi"("Name(\"\" to use uuid) in"=w213) -> ("Error out"=w211:errorcluster, "New State Notifier Event"=w212:refnum<user-event>)  [unwired: 9 in]
        n58 = register-events(error in=w211, w212) -> (reference out=w214:refnum<event-registration>, error out=w210:errorcluster)  [unwired: 1 in]
      }
      frame "Events: Unregister" {
        n59 = Unregister For Events(event registration refnum=w217, error in=w221) -> (error out=w218:errorcluster)
      }
      frame "---------- UI ----------" {
        n60 = call <vilib>:"Add State(s) to Queue__JKI_lib_State_Machine.vi"("State(s) in (\"\")"=w226) -> ("States Out"=w225:string)  [unwired: 14 in]
      }
      frame "UI: Initialize" {
        n61 = call <vilib>:"Add State(s) to Queue__JKI_lib_State_Machine.vi"("State(s) in (\"\")"=w231) -> ("States Out"=w230:string)  [unwired: 14 in]
      }
      frame "UI: Cursor Set" {
        # "Argument"
        n62 = disable-structure "Conditional Disable Structure" shown="Default" {
          disable-tunnel: w235 -> [w241 w246]
          disable-tunnel: [w240 w246] -> w234
          disable-tunnel: w233 -> [w239 _]
          frame condition #0 (active) {
            n63 = case shown="\"Busy\"" w239 {
              tunnel: w241 -> [w243 w245]
              tunnel: [w242 w244] -> w240
              frame "Idle", Default {
                n64 = call <vilib>:"Unset Busy.vi"("error in (no error)"=w243) -> ("error out"=w242:errorcluster)  [unwired: 10 in]
              }
              frame "Busy" {
                n65 = call <vilib>:"Set Busy.vi"("error in (no error)"=w245) -> ("error out"=w244:errorcluster)  [unwired: 9 in, 1 out]
              }
            }
          }
          frame condition #1 {
          }
        }
        n66 = call <vilib>:"Add State(s) to Queue__JKI_lib_State_Machine.vi"("State(s) in (\"\")"=w238) -> ("States Out"=w237:string)  [unwired: 14 in]
      }
      frame "UI: Front Panel State" {
        # "Argument"
        n67 = Unbundle By Name(w250) -> ("Core.Current VI Reference"=w249:refnum<vi>)
        n68 = case shown="\"Hidden\", \"Hide\"" w248 {
          tunnel: w252 -> [w260 w275 w286 w299 w312]
          tunnel: [w262 w276 w288 w301 w314] -> w251
          tunnel: w249 -> [w261 w273 w287 w300 w313]
          frame "Open", "Standard", Default {
            w255 = T2."Standard" ("State")
            n69 = property class="VI"(reference=w261, error in=w260) -> (reference out=w258:refnum<vi>, error out=w259:errorcluster, "FP.State"=w257:T2)
            n70 = Not Equal?(x=w257, y=w255) -> (x != y?=w256:bool)
            n71 = case shown="True" w256 {
              tunnel: [w266 w268] -> w262
              tunnel: w259 -> [w265 w268]
              tunnel: w258 -> [w264 _]
              tunnel: w255 -> [w263 _]
              frame True {
                n72 = invoke class="VI" method="FP.Open"(reference=w264, error in=w265, "Activate"=TRUE, "State"=w263) -> (error out=w266:errorcluster)  [unwired: 1 in, 4 out]
              }
              frame False {
              }
            }
          }
          frame "Close", "Closed" {
            n73 = property class="VI"(reference=w273, error in=w275) -> (reference out=w272:refnum<vi>, error out=w274:errorcluster, "FP.State"=w270:T2)
            n74 = Not Equal?(x=w270, y=T2."Closed" ("Front Panel Window:State")) -> (x != y?=w269:bool)
            n75 = case shown="True" w269 {
              tunnel: [w277 w280] -> w276
              tunnel: w274 -> [w277 w279]
              tunnel: w272 -> [_ w278]
              frame False {
              }
              frame True {
                n76 = invoke class="VI" method="FP.Close"(reference=w278, error in=w279) -> (error out=w280:errorcluster)  [unwired: 1 in, 2 out]
              }
            }
          }
          frame "Hidden", "Hide" {
            w281 = T2."Hidden" ("State")
            n77 = property class="VI"(reference=w287, error in=w286) -> (reference out=w284:refnum<vi>, error out=w285:errorcluster, "FP.State"=w283:T2)
            n78 = Not Equal?(x=w283, y=w281) -> (x != y?=w282:bool)
            n79 = case shown="True" w282 {
              tunnel: [w292 w293] -> w288
              tunnel: w285 -> [w291 w293]
              tunnel: w284 -> [w290 _]
              tunnel: w281 -> [w289 _]
              frame True {
                n80 = invoke class="VI" method="FP.Open"(reference=w290, error in=w291, "State"=w289) -> (error out=w292:errorcluster)  [unwired: 2 in, 4 out]
              }
              frame False {
              }
            }
          }
          frame "Minimize", "Minimized" {
            w294 = T2."Minimized" ("State")
            n81 = property class="VI"(reference=w300, error in=w299) -> (reference out=w297:refnum<vi>, error out=w298:errorcluster, "FP.State"=w296:T2)
            n82 = Not Equal?(x=w296, y=w294) -> (x != y?=w295:bool)
            n83 = case shown="False" w295 {
              tunnel: [w305 w306] -> w301
              tunnel: w298 -> [w304 w306]
              tunnel: w297 -> [w303 _]
              tunnel: w294 -> [w302 _]
              frame True {
                n84 = invoke class="VI" method="FP.Open"(reference=w303, error in=w304, "State"=w302) -> (error out=w305:errorcluster)  [unwired: 2 in, 4 out]
              }
              frame False {
              }
            }
          }
          frame "Maximize", "Maximized" {
            w307 = T2."Maximized" ("State")
            n85 = property class="VI"(reference=w313, error in=w312) -> (reference out=w310:refnum<vi>, error out=w311:errorcluster, "FP.State"=w309:T2)
            n86 = Not Equal?(x=w309, y=w307) -> (x != y?=w308:bool)
            n87 = case shown="True" w308 {
              tunnel: [w318 w319] -> w314
              tunnel: w311 -> [w317 w319]
              tunnel: w310 -> [w316 _]
              tunnel: w307 -> [w315 _]
              frame True {
                n88 = invoke class="VI" method="FP.Open"(reference=w316, error in=w317, "State"=w315) -> (error out=w318:errorcluster)  [unwired: 2 in, 4 out]
              }
              frame False {
              }
            }
          }
        }
        n89 = call <vilib>:"Add State(s) to Queue__JKI_lib_State_Machine.vi"("State(s) in (\"\")"=w254) -> ("States Out"=w253:string)  [unwired: 14 in]
      }
      frame "---------- Macro ----------" {
        n90 = call <vilib>:"Add State(s) to Queue__JKI_lib_State_Machine.vi"("State(s) in (\"\")"=w324) -> ("States Out"=w323:string)  [unwired: 14 in]
      }
      frame "Macro: Initialize" {
        w326 = "Data: Initialize\nInitialize Core Data\nEvents: Register\nUI: Initialize\nUI: Front Panel State >> Open"  # Data: Initialize Initialize Core Data Events: Register UI: Initialize UI: Front Panel State >> Open
        n91 = call <vilib>:"Add State(s) to Queue__JKI_lib_State_Machine.vi"("State(s) in Front (\"\")"=w326, "State(s) in (\"\")"=w330) -> ("States Out"=w329:string)  [unwired: 13 in]
      }
      frame "Macro: Exit" {
        n92 = Unbundle By Name(w339) -> ("Core.Close Panel on Exit?"=w338:bool)
        n93 = Select(t="UI: Front Panel State >> Close", s=w338, f="") -> (s? t:f=w335:string)
        n94 = call <vilib>:"Add State(s) to Queue__JKI_lib_State_Machine.vi"("State(s) in Front (\"\")"="//Exit Sub-Modules ", "State(s) in (\"\")"=w335, "State(s) at Back (\"\")"="Data: Cleanup\nEvents: Unregister\nExit") -> ("States Out"=w333:string)  [unwired: 12 in]
        n95 = call <vilib>:"Add State(s) to Queue__JKI_lib_State_Machine.vi"("State(s) in Front (\"\")"=w333, "State(s) in (\"\")"=w342) -> ("States Out"=w341:string)  [unwired: 13 in]
      }
      frame "---------- API ----------" {
      }
      frame "API: API1" {
        n96 = call <userlib>:"CSM - Convert HexStr to Data.vi"("HEX String"=w347) -> ()  [unwired: 7 in, 2 out]
      }
      frame "API: API2" {
      }
      frame "asdfasd" {
      }
      frame "---------- Action ----------" {
        n97 = call <vilib>:"Add State(s) to Queue__JKI_lib_State_Machine.vi"("State(s) in Front (\"\")"="JUr‚ÑS\u0004\\¹pÑS" ("State(s) in Front (\"\")"), "State(s) in (\"\")"=w366) -> ("States Out"=w365:string)  [unwired: 13 in]
      }
      frame "Action: action1" {
        n98 = call "Convert API String Arguments to Data.vim"("Type"="CSM" ("Name(\"\" to use uuid)"), "String"=w368) -> ()  [unwired: 6 in, 2 out]
        n99 = call <vilib>:"Add State(s) to Queue__JKI_lib_State_Machine.vi"("State(s) in (\"\")"=w373) -> ("States Out"=w372:string)  [unwired: 14 in]
      }
      frame "Action: action2" {
        n100 = call <vilib>:"Add State(s) to Queue__JKI_lib_State_Machine.vi"("State(s) in (\"\")"=w378) -> ("States Out"=w377:string)  [unwired: 14 in]
      }
    }
  }
  n101 = control-ref of="Current VI Reference"() -> (w14:refnum<vi>)
  n102 = call-poly "CSM-Helper API.vi"("VI"=w14) -> ("error out"=w10:errorcluster, "CSM-Helper.lvclass"=w11:refnum<class "CSM-Helper.lvclass">)  [unwired: 9 in]
  n103 = control-ref of="Current VI Reference"() -> (w1:refnum<vi>)
  n104 = call-poly "CSM-Helper API.vi"("error in (no error)"=w10, "CSM-Helper in"=w11) -> ("error out"=w8:errorcluster, "CSM-Helper out"=w9:refnum<class "CSM-Helper.lvclass">)  [unwired: 7 in, 1 out]
  n105 = call <vilib>:"Traverse for GObjects.vi"("Traverse Target"=TRef_TravTarget."BD", "Class Name"="SubVI", "VI Refnum"=w1) -> ("error out"=w2:errorcluster, "References"=w5:refnum<vi>[])  [unwired: 5 in, 2 out]
  n106 = for {
    tunnel: w5 -> [w386] mode=indexing
    tunnel: [w385] -> w6 mode=indexing if=w380
    tunnel: w2 -> [w379]
    w383 = refnum<vi> refnum  # SubVI
    n107 = To More Specific Class(target class=w383, reference=w386, error in=w379) -> (specific class reference=w384:refnum<vi>, error out=w382:errorcluster)
    n108 = property class="SubVI"(reference=w384, error in=w382) -> (error out=w381:errorcluster, "VIPath"=w385:path)  [unwired: 1 out]
    n109 = Not(x=w381) -> (.not. x?=w380:bool)
  }
  "Array" <- w6
  n110 = call-poly "CSM-Helper API.vi"("error in (no error)"=w8, "CSM-Helper in"=w9) -> ("error out"=w7:errorcluster)  [unwired: 8 in, 1 out]
  n111 = call <userlib>:"CSM - Send Message and Wait for Reply.vi"("Error In (no error)"=w7, "Target Module"="CSM", "State"="Macro: Exit") -> ()  [unwired: 6 in, 3 out]
